vi "Get Scaled FP to Pic File.vi"(6 "选择文件类型":enum16{"PNG", "JPG", "BMP"}(ring), 7 "仅可见区域":bool, 8 "错误输入（无错误）":errorcluster, 9 "图片文件存储路径":path, 10 "图像参数":cluster{"图像深度":i32, "最大宽度":i32, "最大高度":i32}={"图像深度"=8, "最大宽度"=0, "最大高度"=0} {"图像深度" items=["1位、黑白"=1, "4位、16色"=4, "8位、256色"=8, "24位、真彩色"=24]}, 11 "VI Ref":refnum<vi>) -> (0 "错误输出":errorcluster)   [LabVIEW 2012, in "VIRef.lvlib"]
uses:
  VIRef.lvlib
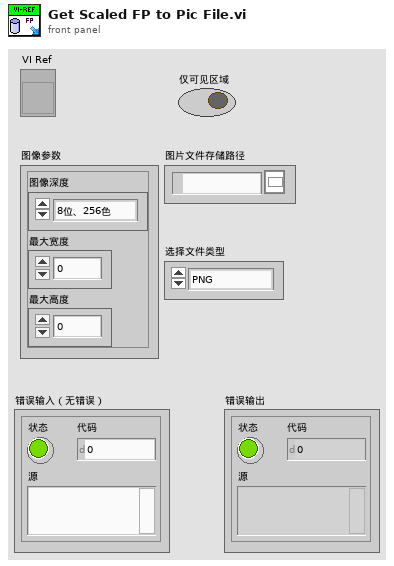
[diagram p1: front panel]
types:
  T1 = typedef "imagedata.ctl" = cluster{"image type":i32, "image depth":i32, "image":u8[], "mask":u8[], "colors":u32[], "Rectangle":cluster{"left":i16, "top":i16, "right":i16, "bottom":i16}}
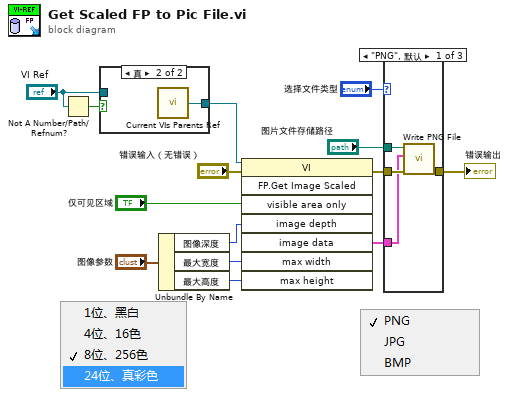
[diagram p0: block diagram]
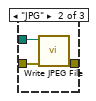
[diagram p2: hidden frame]
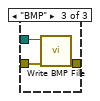
[diagram p3: hidden frame]
diagram:
  n1 = Not A Number/Path/Refnum?(number/path/refnum="VI Ref") -> (NaN/Path/Refnum?=w14:bool)
  n2 = case shown="真" w14 {
    tunnel: [w15 w16] -> w12
    tunnel: "VI Ref" -> [w15 _]
    frame False {
    }
    frame True {
      n3 = call "Current VIs Parents Ref.vi"() -> ("Calling VI's Reference"=w16:refnum<vi>)  [unwired: 2 in]
    }
  }
  n4 = Unbundle By Name("图像参数") -> ("图像深度"=w5:i32, "最大宽度"=w4:i32, "最大高度"=w3:i32)
  n5 = invoke class="VI" method="FP.Get Image Scaled"(reference=w12, error in="错误输入（无错误）", "visible area only"="仅可见区域", "image depth"=w5, "max width"=w4, "max height"=w3) -> (error out=w7:errorcluster, "image data"=w1:T1)  [unwired: 2 in, 6 out]
  n6 = case shown="\"PNG\", 默认" "选择文件类型" {
    tunnel: "图片文件存储路径" -> [w18 w21 w24]
    tunnel: w7 -> [w20 w23 w26]
    tunnel: [w19 w22 w25] -> w6
    tunnel: w1 -> [w17 _ _]
    frame "PNG", Default {
      n7 = call <vilib>:"Write PNG File.vi"("error in (no error)"=w20, "image data"=w17, "path to PNG file"=w18) -> ("error out"=w19:errorcluster)  [unwired: 7 in, 1 out]
    }
    frame "JPG" {
      n8 = call <vilib>:"Write JPEG File.vi"("error in (no error)"=w23, "path to JPEG file"=w21) -> ("error out"=w22:errorcluster)  [unwired: 8 in, 1 out]
    }
    frame "BMP" {
      n9 = call <vilib>:"Write BMP File.vi"("error in (no error)"=w26, "path to BMP file"=w24) -> ("error out"=w25:errorcluster)  [unwired: 8 in, 1 out]
    }
  }
  "错误输出" <- w6
